vi "Init OLED.vi"(8 "error in (no error)":errorcluster, 11 "64x128 I2C OLED SSD1315 in":refnum<class "64x128 I2C OLED SSD1315.lvclass">) -> (0 "error out":errorcluster, 2 "2D Picture":picture, 3 "64x128 I2C OLED SSD1315 out":refnum<class "64x128 I2C OLED SSD1315.lvclass">)   [LabVIEW 2020, in "CTI-Peripheral.lvlib" / "64x128 I2C OLED SSD1315.lvclass"]
uses:
  64x128 I2C OLED SSD1315.lvclass
  64x128 I2C OLED SSD1315.lvclass/64x128 I2C OLED SSD1315.ctl
  CTI/I2C Connection/I2C Connection.lvclass/I2C Connection.ctl
  <vilib>/Utility/High Resolution Relative Seconds.vi
  InitialiseOLED.vi
  CTI/Session/I2C Write Data.vi
  CTI/I2C Connection/I2C Connection.lvclass
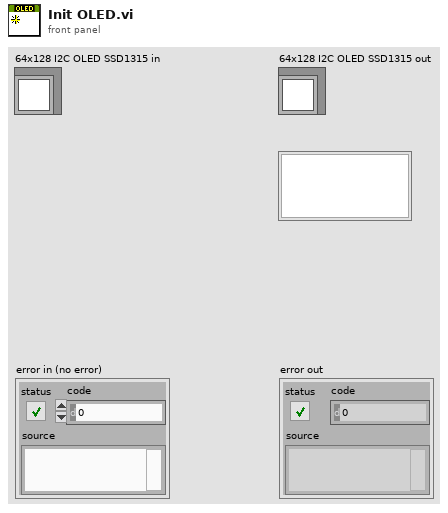
[diagram p1: front panel]
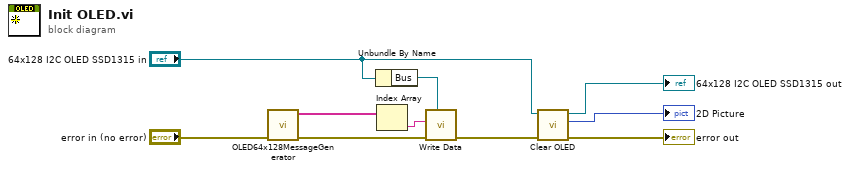
[diagram p0: block diagram]
diagram:
  n1 = call-poly "OLED64x128MessageGenerator.vi"("error in (no error)"="error in (no error)") -> ("error out"=w9:errorcluster, "Messages"=w7:string[])  [unwired: 9 in]
  n2 = Unbundle By Name("64x128 I2C OLED SSD1315 in") -> ("Bus"=w10:refnum<class "I2C Connection.lvclass">)
  n3 = Index Array(array=w7) -> (element=w1:string)  [unwired: 1 in]
  n4 = call "Write Data.vi"("I2C Connection"=w10, "error in (no error)"=w9, "Data"=w1) -> ("error out"=w6:errorcluster)  [unwired: 8 in]
  n5 = call "Clear OLED.vi"("error in (no error)"=w6, "64x128 I2C OLED SSD1315 in"="64x128 I2C OLED SSD1315 in") -> ("error out"=→"error out":errorcluster, "2D Picture"=→"2D Picture":picture, "64x128 I2C OLED SSD1315 out"=→"64x128 I2C OLED SSD1315 out":refnum<class "64x128 I2C OLED SSD1315.lvclass">)  [unwired: 7 in]
